vi "Init Rx Conversion Resources.vi"(8 "error in (no error)":errorcluster, 11 "Rx Loop Data":T1) -> (0 "error out":errorcluster, 3 "Rx Loop Data out":T1)   [LabVIEW 2016, in "UDP-Custom-Device Engine.lvlib"]
uses:
  UDP-Custom-Device Engine.lvlib
  Rx Loop Data.ctl
  <vilib>/NI Veristand/VeriStand Data/Library/Byte Buffer/Byte Buffer.lvclass
  <vilib>/NI/NIVS Inline Async API/_Data Access Engine/Data Access Engine/Types/Write.DVR.ctl
  <vilib>/NI/NIVS Inline Async API/_Data Access Engine/Access Type Classes/Write/Write.lvclass
  <vilib>/NI Veristand/VeriStand Data/Library/Typedefs/Typedefs.Data Types.ctl
  Data Conversion Config.ctl
  <vilib>/NI Veristand/VeriStand Data/Library/Byte Buffer/Byte Buffer.Mapping.ctl
  Shared/Header Details.ctl
  <vilib>/NI Veristand/VeriStand Data/Library/Byte Buffer/Byte Buffer.Mapping.Create (Channel Pointer).vi
  <vilib>/NI Veristand/VeriStand Data/Library/Utilities/Utilities.Sizeof.Array.vi
  <vilib>/NI Veristand/VeriStand Data/Library/Utilities/Utilities.Sizeof.Scalar.vi
  <vilib>/NI Veristand/VeriStand Data/Library/VeriStand Data.lvlib
  <vilib>/NI/NIVS Inline Async API/_Data Access Engine/Data Access Engine/Data Access Engine.lvclass
  Shared/UDP-Custom-Device Shared.lvlib
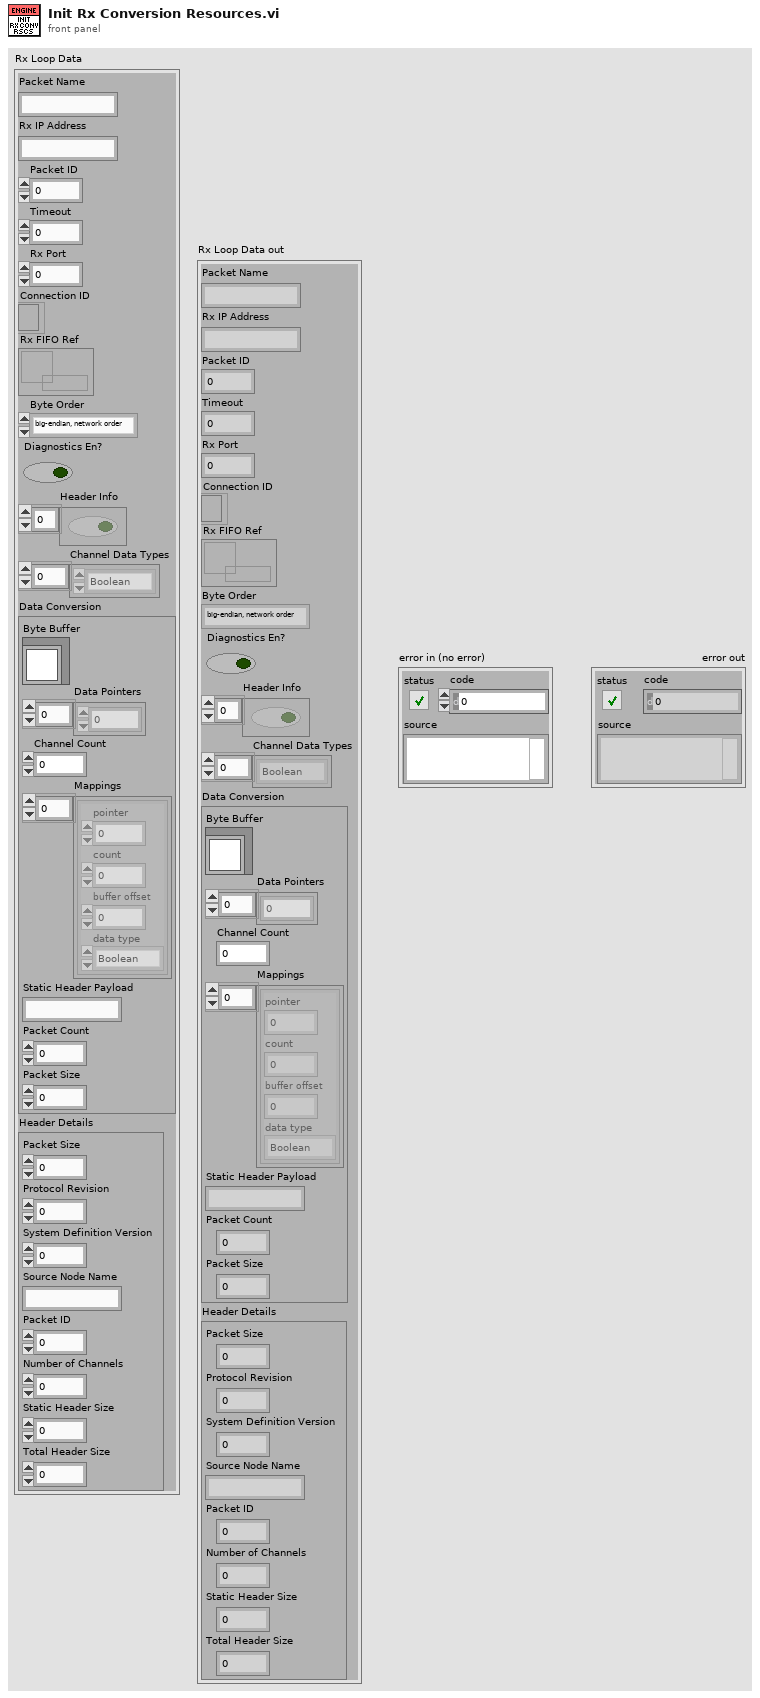
[diagram p1: front panel]
types:
  T1 = typedef "UDP-Custom-Device Engine.lvlib/Rx Loop Data.ctl" = cluster{"Packet Name":string, "Rx IP Address":string, "Packet ID":i32, "Timeout":i32, "Rx Port":i32, "Connection ID":refnum<k16>, "Rx FIFO Ref":T2, "Byte Order":enum16{"big-endian, network order", "native, host order", "little-endian"}, "Diagnostics En?":bool, "Header Info":bool[], "Channel Data Types":T3[], "Data Conversion":T4, "Header Details":T6}
  T2 = typedef "Data Access Engine.lvlib/Data Access Engine.lvclass/Write.DVR.ctl" = refnum<data-value>
  T3 = typedef "VeriStand Data.lvlib/Typedefs.Data Types.ctl" = enum16{"Boolean", "Single", "Double", "I8", "I16", "I32", "I64", "U8", "U16", "U32", "U64"}
  T4 = typedef "UDP-Custom-Device Engine.lvlib/Data Conversion Config.ctl" = cluster{"Byte Buffer":refnum<class "Byte Buffer.lvclass">, "Data Pointers":u64[], "Channel Count":i32, "Mappings":T5[], "Static Header Payload":string, "Packet Count":dbl, "Packet Size":i32}
  T5 = typedef "VeriStand Data.lvlib/Byte Buffer.lvclass/Byte Buffer.Mapping.ctl" = cluster{"pointer":u64, "count":i32, "buffer offset":i32, "data type":T3}
  T6 = typedef "UDP-Custom-Device Shared.lvlib/Header Details.ctl" = cluster{"Packet Size":u16, "Protocol Revision":u8, "System Definition Version":u64, "Source Node Name":string, "Packet ID":u32, "Number of Channels":u32, "Static Header Size":u16, "Total Header Size":u16}
  T7 = enum16{"big-endian, network order", "native, host order", "little-endian"}
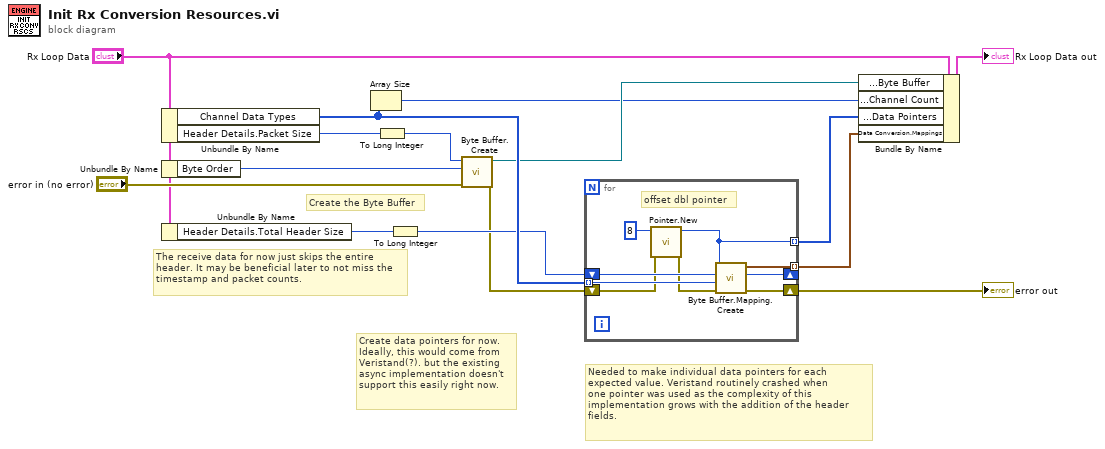
[diagram p0: block diagram]
diagram:
  # "Needed to make individual data pointers for each\nexpected value. Veristand routinely crashed when\none pointer was used as the complexity of this\nimplementation grows with the addition of the header\nfields."
  # "Create data pointers for now.\nIdeally, this would come from\nVeristand(?). but the existing\nasync implementation doesn't\nsupport this easily right now."
  # "The receive data for now just skips the entire\nheader. It may be beneficial later to not miss the\ntimestamp and packet counts."
  # "Create the Byte Buffer"
  n1 = Unbundle By Name("Rx Loop Data") -> ("Channel Data Types"=w13:T3[], "Header Details.Packet Size"=w8:u16)
  n2 = Unbundle By Name("Rx Loop Data") -> ("Byte Order"=w15:T7)
  n3 = Unbundle By Name("Rx Loop Data") -> ("Header Details.Total Header Size"=w5:u16)
  n4 = Array Size(array=w13) -> (size(s)=w3:i32)
  n5 = To Long Integer(number=w8) -> (32bit integer=w7:i32)
  n6 = To Long Integer(number=w5) -> (32bit integer=w4:i32)
  n7 = call <vilib>:"Byte Buffer.Create.vi"("error in (no error)"="error in (no error)", "byte order (big-endian)"=w15, "size"=w7) -> ("error out"=w2:errorcluster, "Byte Buffer"=w11:refnum<class "Byte Buffer.lvclass">)  [unwired: 7 in]
  n8 = for {
    tunnel: [w24] -> w10 mode=indexing
    tunnel: w13 -> [w22] mode=indexing
    shift-right: [w23] -> w9
    shift-left: w2 -> [w19]
    shift-right: [w21] -> _
    shift-left: w4 -> [w20]
    tunnel: [w16] -> w1 mode=indexing
    # "offset dbl pointer"
    n9 = call <vilib>:"Pointer.New.vi"("error in (no error)"=w19, "size in bytes"=8 ("x")) -> ("error out"=w18:errorcluster, "pointer"=w16:u64)  [unwired: 8 in]
    n10 = call-poly <vilib>:"Byte Buffer.Mapping.Create.vi"("error in (no error)"=w18, "data type"=w22, "buffer offset"=w20, "Channel Pointer"=w16) -> ("error out"=w23:errorcluster, "new buffer offset"=w21:i32, "mapping"=w24:T5)  [unwired: 5 in]
  }
  "error out" <- w9
  n11 = Bundle By Name(cluster="Rx Loop Data", "Data Conversion.Byte Buffer"=w11, "Data Conversion.Channel Count"=w3, "Data Conversion.Data Pointers"=w1, "Data Conversion.Mappings"=w10) -> (→"Rx Loop Data out":T1)
